vi "Create Event.vi"(9 "Event":refnum<class "Event.lvclass">, 10 "Self Event Alias":string, 11 "Create Event in":refnum<class "Create Event.lvclass">) -> (3 "Create Event out":refnum<class "Create Event.lvclass">)   [LabVIEW 2021, in "Create Event Msg Strategy.lvlib" / "Create Event.lvclass"]
uses:
  Create Event.lvclass
  jettl/Event/Event.lvclass
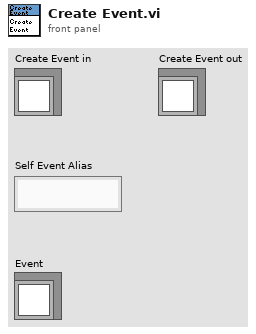
[diagram p1: front panel]
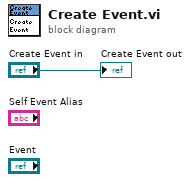
[diagram p0: block diagram]
diagram:
  "Create Event out" <- "Create Event in"
